vi "loops.vi"() -> ()   [LabVIEW 2022 SP3]
panel:
  out "Numeric":dbl
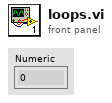
[diagram p1: front panel]
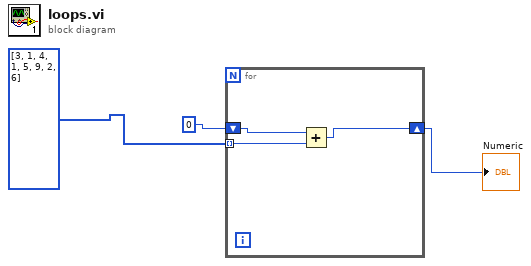
[diagram p0: block diagram]
diagram:
  n1 = for {
    tunnel: i32[] [3, 1, 4, 1, 5, 9, 2, 6] -> [w4] mode=indexing
    shift-right: [w6] -> w2
    shift-left: 0 -> [w5]
    n2 = Add(x=w5, y=w4) -> (x+y=w6:i32)
  }
  "Numeric" <- w2
